vi "set_PV.vi"(0 "HGF_NetworkVisitor":refnum<class "HGF_NetworkVisitor.lvclass">, 2 "HGF_PVSubscriber":refnum<class "HGF_PVSubscriber.lvclass">, 5 "error in (no error)":errorcluster) -> (14 "dup HGF_NetworkVisitor":refnum<class "HGF_NetworkVisitor.lvclass">, 19 "error out":errorcluster)   [LabVIEW 2014, in "HGF_BaseClasses.lvlib" / "HGF_NetworkVisitor.lvclass"]
doc: "Set Provess Variable."
uses:
  HGF_NetworkVisitor.lvclass
  HGF_PVSubscriber/HGF_PVSubscriber.lvclass
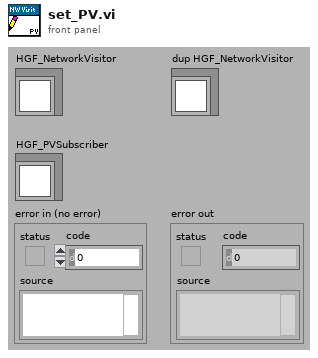
[diagram p1: front panel]
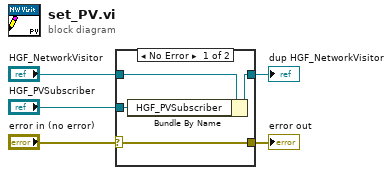
[diagram p0: block diagram]
diagram:
  n1 = case shown="No Error" "error in (no error)" {
    selector: "error in (no error)" -> [w9 w10]
    tunnel: [w9 w10] -> w4
    tunnel: [w7 w11] -> w2
    tunnel: "HGF_NetworkVisitor" -> [w8 w11]
    tunnel: "HGF_PVSubscriber" -> [w6 _]
    frame No Error {
      n2 = Bundle By Name(cluster=w8, "HGF_PVSubscriber"=w6) -> (w7:refnum<class "HGF_NetworkVisitor.lvclass">)
    }
    frame Error {
    }
  }
  "error out" <- w4
  "dup HGF_NetworkVisitor" <- w2
